vi "DrawArms.vi"(0 "Stage in":refnum<vi>, 1 "Params":T2={"Line width"=0.1, "Line Color"=4376575, "Axes?"=TRUE}, 2 "Start":T1=[[1.0, 0.0, 0.0, 0.0], [0.0, 1.0, 0.0, 0.0], [0.0, 0.0, 1.0, 0.0], [0.0, 0.0, 0.0, 1.0]], 3 "End":T1) -> (5 "Stage out":refnum<vi>, 6 "End Out":T1)   [LabVIEW 2018]
uses:
  <vilib>/Analysis/Matrix/Datatypes/RealMatrix.ctl
  <vilib>/Analysis/Matrix/NI_Matrix.lvlib
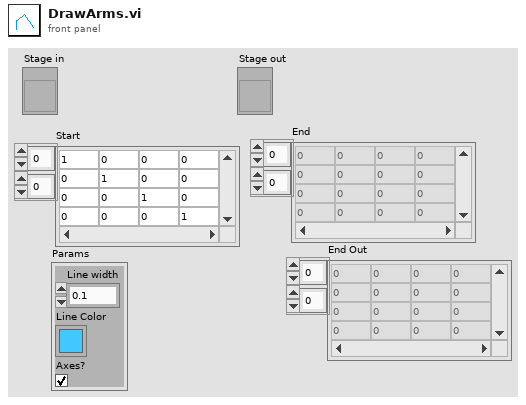
[diagram p1: front panel]
types:
  T1 = typedef "NI_Matrix.lvlib/RealMatrix.ctl" = dbl[][]
  T2 = cluster{"Line width":sgl, "Line Color":u32, "Axes?":bool}
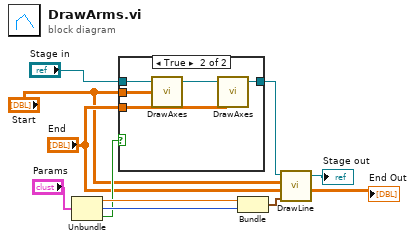
[diagram p0: block diagram]
diagram:
  n1 = Unbundle("Params") -> ("Line width"=w6:sgl, "Line Color"=w5:u32, "Axes?"=w3:bool)
  n2 = case shown="True" w3 {
    tunnel: "Start" -> [_ w16]
    tunnel: [w11 w15] -> w9
    tunnel: "Stage in" -> [w11 w13]
    tunnel: "End" -> [_ w12]
    frame False {
    }
    frame True {
      n3 = call "DrawAxes.vi"("Axes"=w16, "Stage in"=w13) -> ("Stage out"=w14:refnum<vi>)  [unwired: 3 in]
      n4 = call "DrawAxes.vi"("Axes"=w12, "Stage in"=w14) -> ("Stage out"=w15:refnum<vi>)  [unwired: 3 in]
    }
  }
  n5 = Bundle("Line width"=w6, "Line Color"=w5) -> (w4:cluster{"Line width":sgl, "Line Color":u32})  [unwired: 1 in]
  n6 = call "DrawLine.vi"("Params"=w4, "Axes2"="End", "Axes1"="Start", "Stage in"=w9) -> ("Stage out"=→"Stage out":refnum<vi>)  [unwired: 1 in, 1 out]
  "End Out" <- "End"
